vi "Bloch Sphere Model.vi"(9 "Phi":dbl, 10 "Theta":dbl, 11 "Length":dbl) -> (3 "SceneObject out":refnum<vi>)   [LabVIEW 2020]
uses:
  <vilib>/picture/3D Picture Control/Object/Create Object (name).vi
  <vilib>/picture/3D Picture Control/Object/Add Object (no reference).vi
  <vilib>/picture/3D Picture Control/Object/Create Object (drawable).vi
  <vilib>/picture/3D Picture Control/NI_3D Picture Control.lvlib
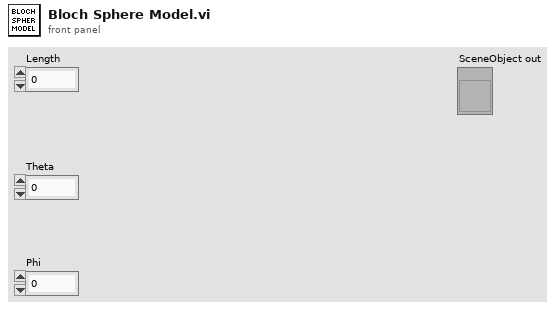
[diagram p1: front panel]
types:
  T1 = enum16{"Inherit Value", "Points", "Wireframe", "Polygons"}
  T2 = enum16{"Inherit Value", "No Culling", "Cull Back Face", "Cull Front Face", "Cull Both Faces"}
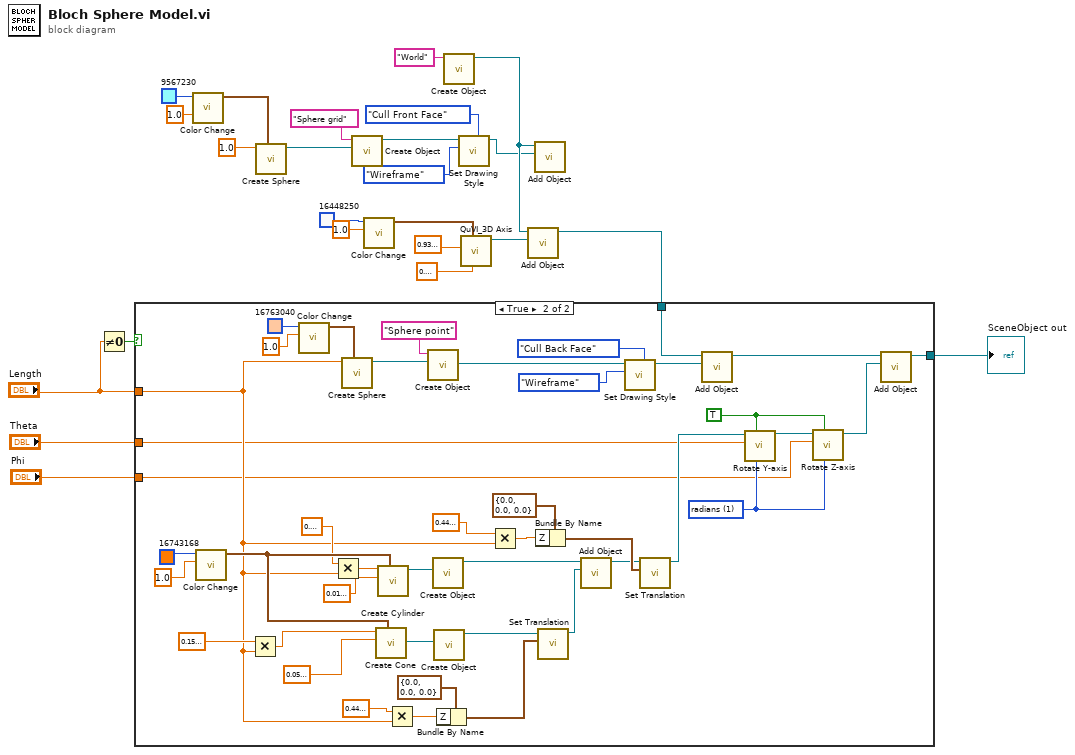
[diagram p0: block diagram]
diagram:
  n1 = Not Equal To 0?(x="Length") -> (x != 0?=w22:bool)
  n2 = call <vilib>:"Color Change.vi"("Alpha"=1.0, "Color"=u32 9567230) -> ("RGBA"=w2:cluster{"R":sgl, "G":sgl, "B":sgl, "A":sgl})  [unwired: 9 in]
  n3 = call <vilib>:"Create Sphere.vi"("Color"=w2, "Radius"=sgl 1.0) -> ("New Sphere Refnum"=w3:refnum<vi>)  [unwired: 8 in, 1 out]
  n4 = call-poly <vilib>:"Create Object.vi"("Geometry"=w3, "Name"="Sphere grid") -> ("Scene:New Object"=w11:refnum<vi>)  [unwired: 8 in, 1 out]
  n5 = call <vilib>:"Color Change.vi"("Alpha"=1.0, "Color"=u32 16448250) -> ("RGBA"=w8:cluster{"R":sgl, "G":sgl, "B":sgl, "A":sgl})  [unwired: 9 in]
  n6 = call-poly <vilib>:"Create Object.vi"("Name"="World") -> ("Scene:New Object"=w20:refnum<vi>)  [unwired: 9 in, 1 out]
  n7 = call <vilib>:"Set Drawing Style.vi"("Face Culling Mode"=T2."Cull Front Face", "Mode"=T1."Wireframe", "Scene Object In"=w11) -> ("Scene Object Out"=w12:refnum<vi>)  [unwired: 7 in, 1 out]
  n8 = call "QuVI_3D Axis.vi"("Character Size"=sgl 0.2, "Color"=w8, "Length"=sgl 0.93) -> ("New Object Refnum"=w9:refnum<vi>)  [unwired: 7 in, 1 out]
  n9 = call-poly <vilib>:"Add Object.vi"("New Object In"=w9, "Scene Object In"=w20) -> ("Scene Object Out"=w21:refnum<vi>)  [unwired: 8 in, 1 out]
  n10 = case shown="True" w22 {
    tunnel: "Length" -> [_ w32]
    tunnel: "Phi" -> [_ w30]
    tunnel: "Theta" -> [_ w29]
    tunnel: w21 -> [w25 w27]
    tunnel: [w25 w26] -> w24
    frame False {
    }
    frame True {
      w42 = u16 1 items=["degree", "radians"] ("angle unit")
      w45 = TRUE ("Relative?")
      n11 = call <vilib>:"Color Change.vi"("Alpha"=1.0, "Color"=u32 16743168) -> ("RGBA"=w55:cluster{"R":sgl, "G":sgl, "B":sgl, "A":sgl})  [unwired: 9 in]
      n12 = Multiply(x=0.15000000596046448 ("Height"), y=w32) -> (x*y=w33:dbl)
      n13 = call <vilib>:"Color Change.vi"("Alpha"=1.0, "Color"=u32 16763040) -> ("RGBA"=w46:cluster{"R":sgl, "G":sgl, "B":sgl, "A":sgl})  [unwired: 9 in]
      n14 = Multiply(x=0.8999999761581421 ("Height"), y=w32) -> (x*y=w36:dbl)
      n15 = call <vilib>:"Create Sphere.vi"("Color"=w46, "Radius"=w32) -> ("New Sphere Refnum"=w66:refnum<vi>)  [unwired: 8 in, 1 out]
      n16 = call <vilib>:"Create Cone.vi"("Color"=w55, "Radius"=sgl 0.05, "Height"=w33) -> ("New Cone Refnum"=w65:refnum<vi>)  [unwired: 7 in, 1 out]
      n17 = call <vilib>:"Create Cylinder.vi"("Color"=w55, "Radius"=sgl 0.02, "Height"=w36) -> ("New Cylinder Refnum"=w64:refnum<vi>)  [unwired: 7 in, 1 out]
      n18 = Multiply(x=0.44999998807907104 ("Z"), y=w32) -> (x*y=w39:dbl)
      n19 = call-poly <vilib>:"Create Object.vi"("Geometry"=w66, "Name"="Sphere point") -> ("Scene:New Object"=w67:refnum<vi>)  [unwired: 8 in, 1 out]
      n20 = call-poly <vilib>:"Create Object.vi"("Geometry"=w64) -> ("Scene:New Object"=w58:refnum<vi>)  [unwired: 9 in, 1 out]
      n21 = call-poly <vilib>:"Create Object.vi"("Geometry"=w65) -> ("Scene:New Object"=w54:refnum<vi>)  [unwired: 9 in, 1 out]
      n22 = Bundle By Name(cluster=cluster{"X":sgl, "Y":sgl, "Z":sgl} {"X"=0.0, "Y"=0.0, "Z"=0.0} ("Translation"), "Z"=w39) -> (w51:cluster{"X":sgl, "Y":sgl, "Z":sgl})
      n23 = Multiply(x=0.44999998807907104 ("Z"), y=w32) -> (x*y=w40:dbl)
      n24 = Bundle By Name(cluster=cluster{"X":sgl, "Y":sgl, "Z":sgl} {"X"=0.0, "Y"=0.0, "Z"=0.0} ("Translation"), "Z"=w40) -> (w59:cluster{"X":sgl, "Y":sgl, "Z":sgl})
      n25 = call <vilib>:"Set Translation.vi"("Translation"=w51, "Scene Object"=w54) -> ("Translated Object"=w53:refnum<vi>)  [unwired: 8 in, 1 out]
      n26 = call-poly <vilib>:"Add Object.vi"("New Object In"=w53, "Scene Object In"=w58) -> ("Scene Object Out"=w57:refnum<vi>)  [unwired: 8 in, 1 out]
      n27 = call <vilib>:"Set Drawing Style.vi"("Face Culling Mode"=T2."Cull Back Face", "Mode"=T1."Wireframe", "Scene Object In"=w67) -> ("Scene Object Out"=w61:refnum<vi>)  [unwired: 7 in, 1 out]
      n28 = call <vilib>:"Set Translation.vi"("Translation"=w59, "Scene Object"=w57) -> ("Translated Object"=w31:refnum<vi>)  [unwired: 8 in, 1 out]
      n29 = call-poly <vilib>:"Add Object.vi"("New Object In"=w61, "Scene Object In"=w27) -> ("Scene Object Out"=w28:refnum<vi>)  [unwired: 8 in, 1 out]
      n30 = call <vilib>:"Rotate Y-axis.vi"("angle unit"=w42, "Relative?"=w45, "angle"=w29, "Scene Object In"=w31) -> ("Scene Object Out"=w44:refnum<vi>)  [unwired: 6 in, 1 out]
      n31 = call <vilib>:"Rotate Z-axis.vi"("angle unit"=w42, "Relative?"=w45, "angle"=w30, "Scene Object In"=w44) -> ("Scene Object Out"=w43:refnum<vi>)  [unwired: 6 in, 1 out]
      n32 = call-poly <vilib>:"Add Object.vi"("New Object In"=w43, "Scene Object In"=w28) -> ("Scene Object Out"=w26:refnum<vi>)  [unwired: 8 in, 1 out]
    }
  }
  "SceneObject out" <- w24
  n33 = call-poly <vilib>:"Add Object.vi"("New Object In"=w12, "Scene Object In"=w20) -> ()  [unwired: 8 in, 2 out]
